vi "Monitor Command.vi"(8 "error in (no error)":errorcluster, 10 "StartStop":bool, 11 "Application Controller in":refnum<class "Application Controller.lvclass">) -> (0 "error out":errorcluster, 3 "Application Controller out":refnum<class "Application Controller.lvclass">)   [LabVIEW 2016, in "Application Controller.lvclass"]
uses:
  Application Controller.lvclass
  Application Controller.lvclass/Application Controller.ctl
  Read Monitor start event.vi
  Read Monitor stop event.vi
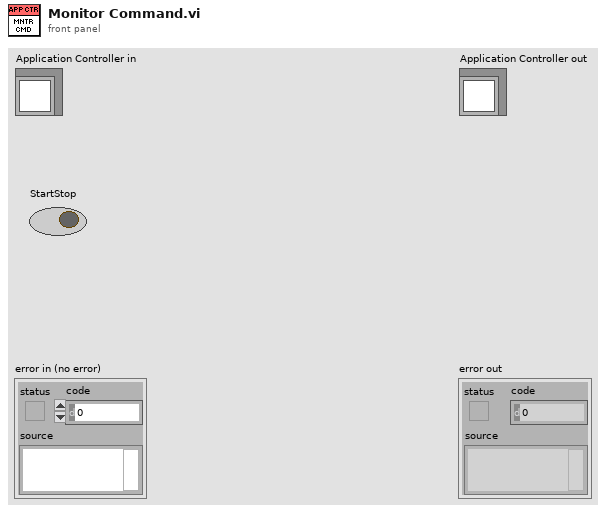
[diagram p1: front panel]
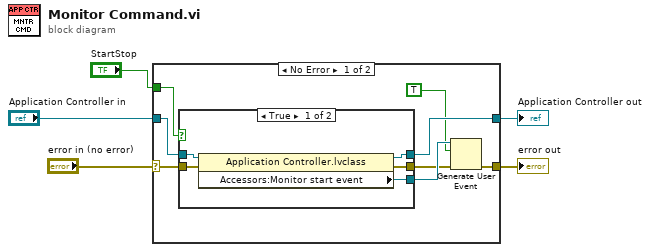
[diagram p0: block diagram]
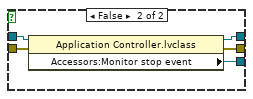
[diagram p2: hidden frame]
diagram:
  n1 = case shown="No Error" "error in (no error)" {
    selector: "error in (no error)" -> [w13 w25]
    tunnel: [w6 w25] -> w4
    tunnel: [w11 w24] -> w2
    tunnel: "Application Controller in" -> [w12 w24]
    tunnel: "StartStop" -> [w10 _]
    frame No Error {
      n2 = case shown="True" w10 {
        tunnel: w13 -> [w18 w23]
        tunnel: w12 -> [w17 w22]
        tunnel: [w16 w21] -> w11
        tunnel: [w15 w20] -> w9
        tunnel: [w14 w19] -> w7
        frame True {
          n3 = property class="Application Controller.lvclass"(reference=w17, error in=w18) -> (reference out=w16:refnum<class "Application Controller.lvclass">, error out=w14:errorcluster, "Accessors:Monitor start event"=w15:refnum<user-event>)
        }
        frame False {
          n4 = property class="Application Controller.lvclass"(reference=w22, error in=w23) -> (reference out=w21:refnum<class "Application Controller.lvclass">, error out=w19:errorcluster, "Accessors:Monitor stop event"=w20:refnum<user-event>)
        }
      }
      n5 = Generate User Event(user event=w9, event data cluster=TRUE, error in=w7) -> (error out=w6:errorcluster)  [unwired: 1 in, 1 out]
    }
    frame Error {
    }
  }
  "error out" <- w4
  "Application Controller out" <- w2
